vi "specs_prodigy.vi"() -> ()   [LabVIEW 2020]
uses:
  Github/ARPEScontrol/subvi/PHOIBOS/DEFINITIONS/DEF_dev_state.ctl
  Github/ARPEScontrol/subvi/PHOIBOS/DEFINITIONS/DEF_dev_type.ctl
panel:
  in  "stop":bool
  in  "ana_mode":T1(ring)=enum."WideAngleMode"
  in  "ana_voltrange":enum16{"3.5kV", "1.5kV", "400V", "100V", "10V"}(ring)=enum."400V"
  in  "phoib_I_2s":dbl=35.0
  in  "phoib_I_1s":dbl=21.0
  in  "phoib_I_6s":dbl=3200.0
  in  "phoib_I_4s":dbl=4.558
  in  "phoib_I_3s":dbl=-10.0
  in  "phoib_I_5s":dbl=1700.0
  in  "phoib_I_7s":dbl=-30.0
  in  "phoib_I_8s":dbl=0.0039
  in  "phoib_I_9s":dbl
  in  "phoib_I_10s":dbl
  out "phoib_I_4":dbl=4.558 caption="Work Function"
  out "phoib_I_5":dbl=1500.0 caption="Detctor Voltage"
  out "phoib_I_6":dbl=3200.0 caption="Screen Voltage"
  out "phoib_I_3":dbl=-10.0 caption="Coil Current"
  out "phoib_I_2":dbl=35.0 caption="Pass Energy"
  out "phoib_I_1":dbl=21.0 caption="Kinetic Energy"
  out "state":T2=1 items=["Off"=-1, "Standby"=0, "On"=1]
  out "phoib_I_7":dbl=-30.0 caption="Conversion Voltage"
  out "phoib_I_8":dbl=0.0039 caption="FD1"
  out "phoib_I_9":dbl caption="Mesh Front"
  out "phoib_I_10":dbl caption="Mesh Back"
  out "phoib_error":errorcluster
  out "phoib_con?":bool caption="PHOIBOS"
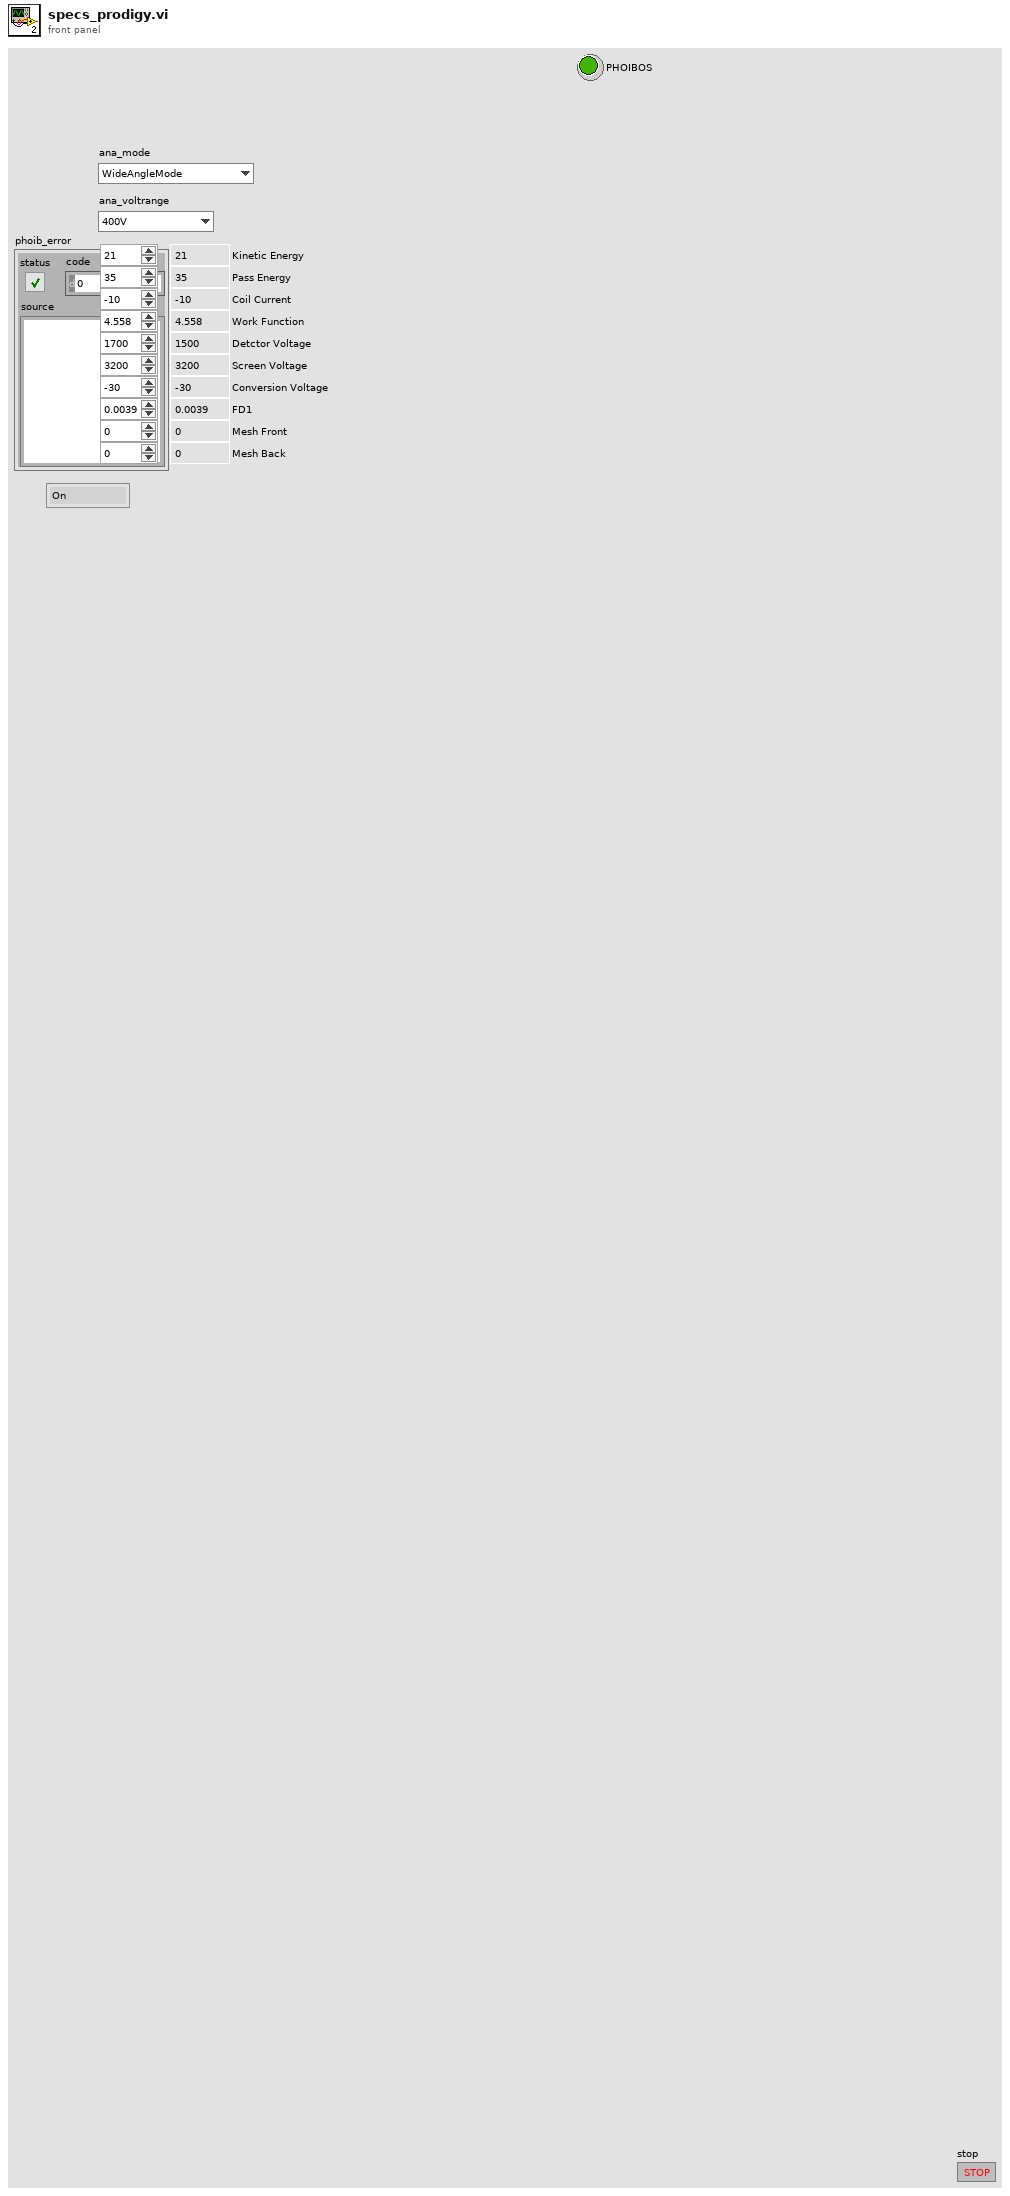
[diagram p1: front panel]
types:
  T1 = enum16{"HighMagnification", "MediumMagnification", "LowMagnification", "HighAngularDispersion", "MediumAngularDispersion", "LowAngularDispersion", "WideAngleMode", "LargeArea", "MediumArea", "SmallArea", "HighMagnification2", "SmallArea2"}
  T2 = typedef "DEF_dev_state.ctl" = i32
  T3 = typedef "DEF_dev_type.ctl" = enum32{"devA (analyzer)", "devD (detector)"}
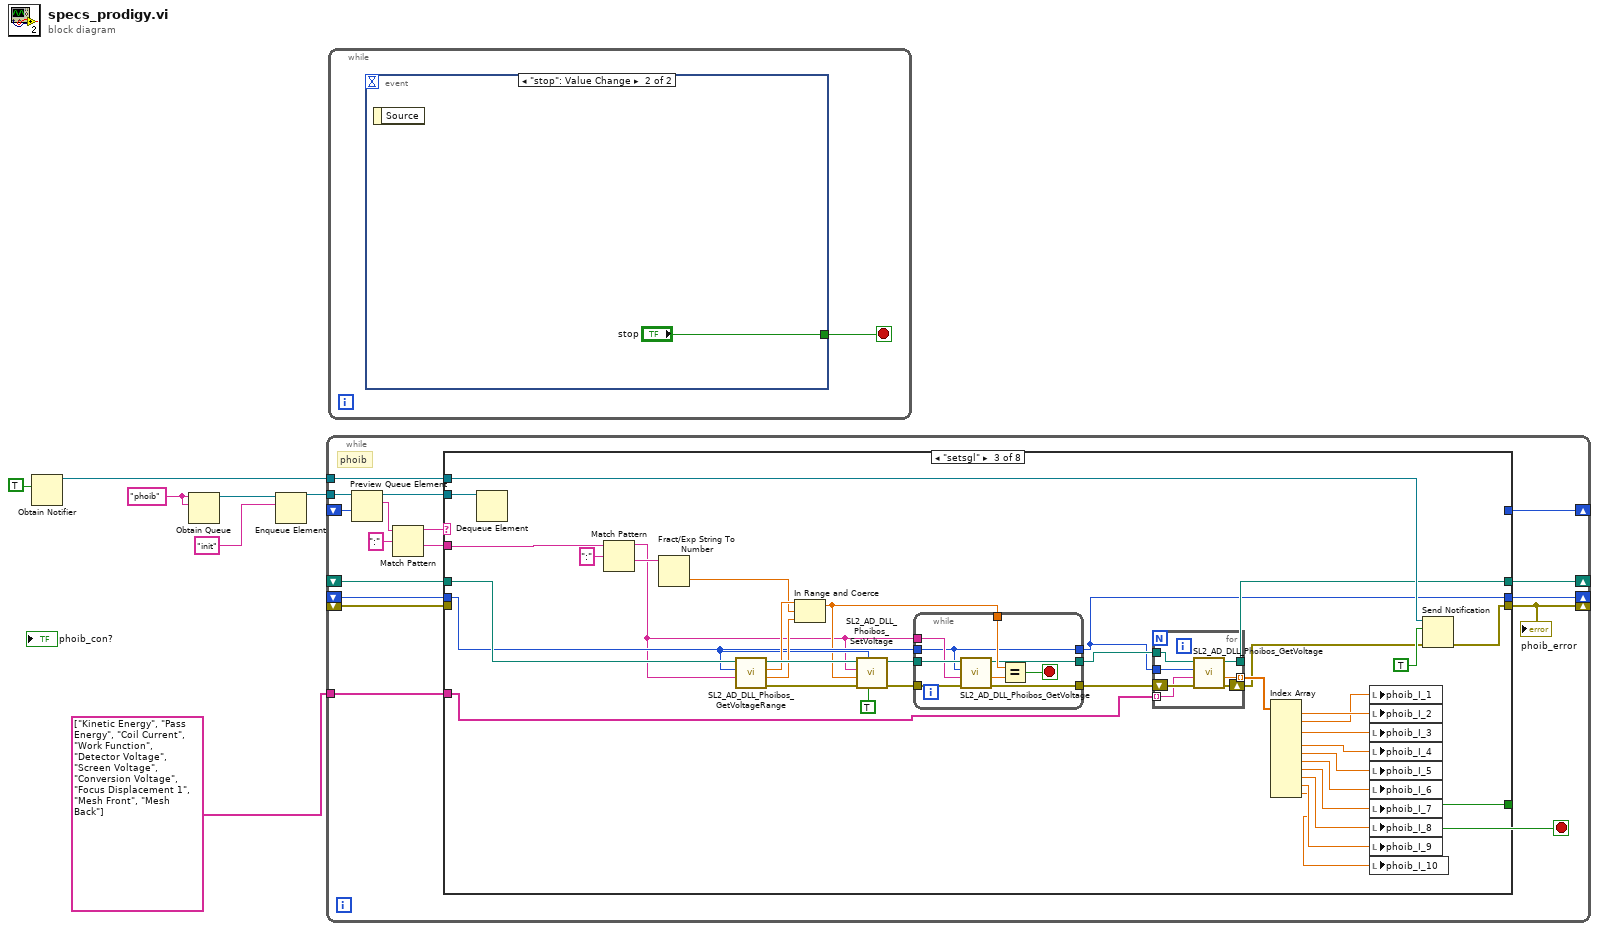
[diagram p0: block diagram]
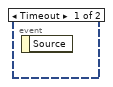
[diagram p2: hidden frame]
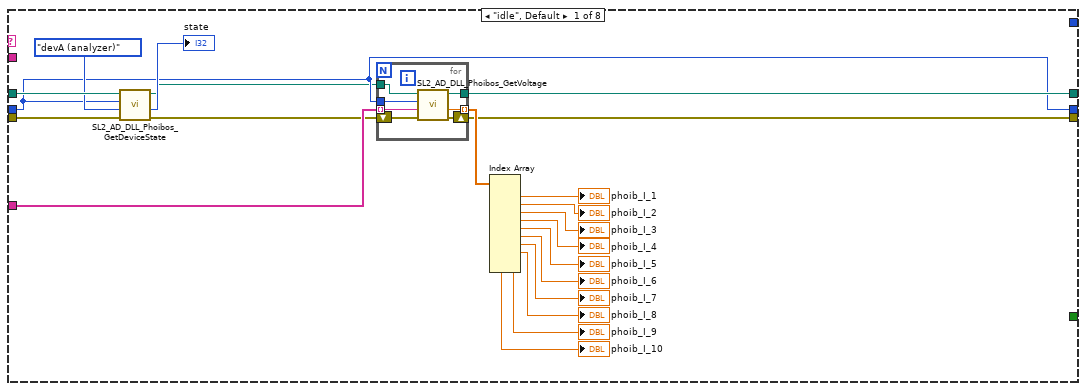
[diagram p3: hidden frame]
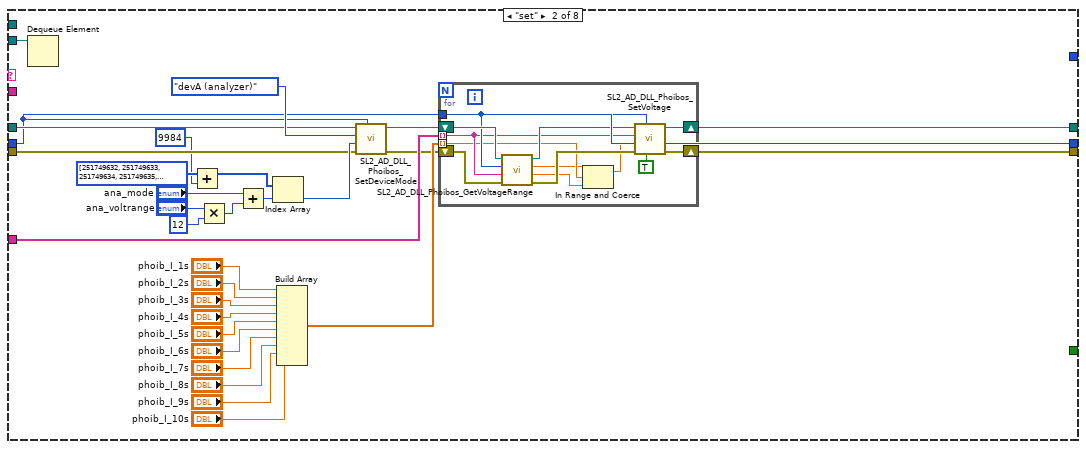
[diagram p4: hidden frame]
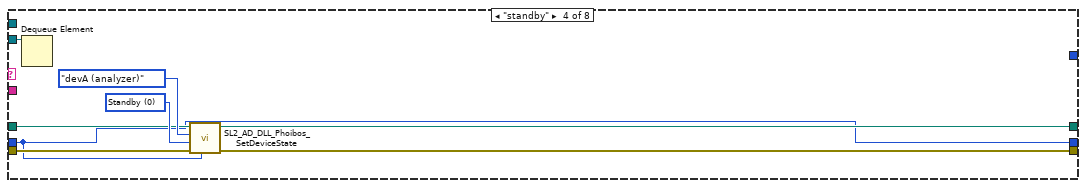
[diagram p5: hidden frame]
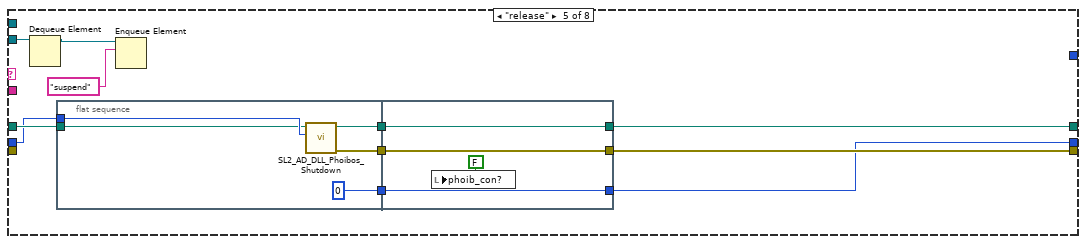
[diagram p6: hidden frame]
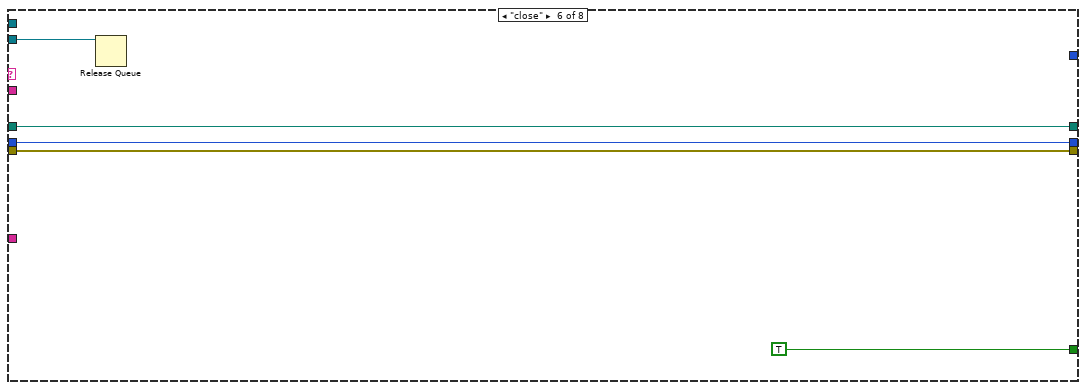
[diagram p7: hidden frame]
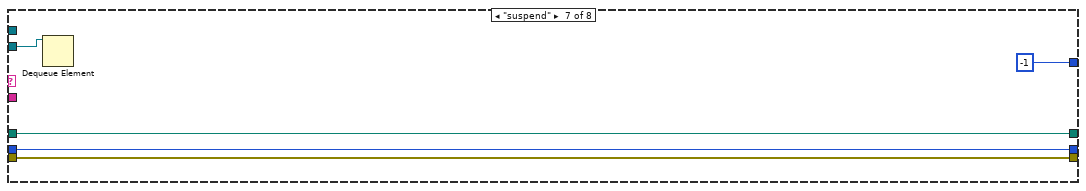
[diagram p8: hidden frame]
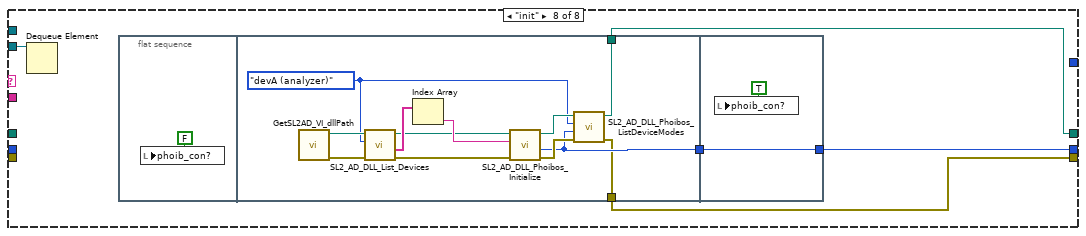
[diagram p9: hidden frame]
diagram:
  w4 = "phoib" ("name (unnamed)")
  n1 = Obtain Notifier(notification data type=TRUE) -> (notifier out=w2:refnum<notifier>)  [unwired: 3 in, 2 out]
  n2 = Obtain Queue(name (unnamed)=w4, element data type=w4) -> (queue out=w7:refnum<queue>)  [unwired: 3 in, 2 out]
  n3 = Enqueue Element(queue=w7, element="init") -> (queue out=w6:refnum<queue>)  [unwired: 2 in, 2 out]
  n4 = while {
    tunnel: w6 -> [w19]
    shift-right: [w8] -> _
    shift-left: _ -> [w17]
    shift-right: [w16] -> _
    shift-left: _ -> [w15]
    shift-right: [w14] -> _
    shift-left: _ -> [w13]
    shift-right: [w12] -> _
    shift-left: _ -> [w11]
    tunnel: string[] ["Kinetic Energy", "Pass Energy", "Coil Current", "Work Function", "Detector Voltage", "Screen Voltage", "Conversion Voltage", "Focus Displacement 1", "Mesh Front", "Mesh Back"] -> [w10]
    tunnel: w2 -> [w9]
    stop <- w18 stop-if-true
    # "phoib"
    n5 = Preview Queue Element(queue=w19, timeout in ms (-1)=w17) -> (queue out=w22:refnum<queue>, element=w23:string)  [unwired: 1 in, 2 out]
    n6 = Match Pattern(string=w23, regular expression=":") -> (before substring=w21:string, after substring=w20:string)  [unwired: 1 in, 2 out]
    n7 = case shown="\"setsgl\"" w21 {
      tunnel: w22 -> [_ w80 w131 w148 w166 w180 w185 w190]
      tunnel: w20 -> [_ _ w96 _ _ _ _ _]
      tunnel: [_ _ _ _ _ TRUE _ _] -> w18
      tunnel: [w34 w82 w101 w151 w164 w178 w184 w187] -> w16
      tunnel: w15 -> [w45 w71 w122 w153 w165 w178 w184 _]
      tunnel: [w33 w81 w117 w150 w163 w176 w182 w186] -> w14
      tunnel: w13 -> [w43 w70 _ w152 _ w176 w182 _]
      tunnel: [w31 w68 w100 w149 w162 w177 w183 w189] -> w12
      tunnel: w11 -> [w31 w68 w120 w149 w161 w177 w183 _]
      tunnel: w10 -> [w32 w61 w98 _ _ _ _ _]
      tunnel: w9 -> [_ _ w116 _ _ _ _ _]
      tunnel: [_ _ _ _ _ _ -1 _] -> w8
      frame "idle", Default {
        n8 = call "SL2_AD_DLL_Phoibos_GetDeviceState.vi"("dll_path"=w45, "pHandle_in"=w31, "dev_type"=DEF_dev_type."devA (analyzer)", "error in"=w43) -> ("path out"=w30:path, "state"=→"state":T2, "error out"=w29:errorcluster)  [unwired: 2 in]
        n9 = for {
          tunnel: w31 -> [w52]
          tunnel: w32 -> [w50] mode=indexing
          tunnel: [w49] -> w42 mode=indexing
          tunnel: [w48] -> w34
          shift-right: [w47] -> w33
          shift-left: w29 -> [w51]
          tunnel: w30 -> [w46]
          n10 = call "SL2_AD_DLL_Phoibos_GetVoltage.vi"("error in"=w51, "voltage_name"=w50, "pHandle"=w52, "dll path in"=w46) -> ("error out"=w47:errorcluster, "value"=w49:dbl, "dll path out"=w48:path)  [unwired: 3 in]
        }
        n11 = Index Array(array=w42) -> (element #1=→"phoib_I_1":dbl, element #2=→"phoib_I_2":dbl, element #3=→"phoib_I_3":dbl, element #4=→"phoib_I_4":dbl, element #5=→"phoib_I_5":dbl, element #6=→"phoib_I_6":dbl, element #7=→"phoib_I_7":dbl, element #8=→"phoib_I_8":dbl, element #9=→"phoib_I_9":dbl, element #10=→"phoib_I_10":dbl)  [unwired: 10 in]
      }
      frame "set" {
        n12 = Dequeue Element(queue=w80) -> ()  [unwired: 2 in, 4 out]
        n13 = Add(x=u32[] [251749632, 251749633, 251749634, 251749635, 251749636, 251749637, 251749638, 251749639, 251749640, 251749641, 251749642, 251749643, 251749644, 251749645, 251749646, 251749647, 251749648, 251749649, 251749650, 251749651, 251749652, 251749653, 251749654, 251749655, 251749656, 251749657, 251749658, 251749659, 251749660, 251749661, 251749662, 251749663, 251749664, 251749665, 251749666, 251749667, 251749668, 251749669, 251749670, 251749671, 251749672, 251749673, 251749674, 251749675, 251749676, 251749677, 251749678, 251749679, 251749680, 251749681, 251749682, 251749683, 251749684, 251749685, 251749686, 251749687, 251749688, 251749689, 251749690, 251749691, 251749692, 251749693, 251749694, 251749695, 251749696] ("modeIDs"), y=9984) -> (x+y=w54:u32[])
        n14 = Multiply(x="ana_voltrange", y=12) -> (x*y=w77:i32)
        n15 = Add(x="ana_mode", y=w77) -> (x+y=w74:i32)
        n16 = Index Array(array=w54, index=w74) -> (element=w72:u32)
        n17 = Build Array("phoib_I_1s", "phoib_I_2s", "phoib_I_3s", "phoib_I_4s", "phoib_I_5s", "phoib_I_6s", "phoib_I_7s", "phoib_I_8s", "phoib_I_9s", "phoib_I_10s") -> (w60:dbl[])
        n18 = call "SL2_AD_DLL_Phoibos_SetDeviceMode.vi"("pHandle"=w68, "error in"=w70, "value"=w72, "dev_type"=DEF_dev_type."devA (analyzer)", "dll path in"=w71) -> ("error out"=w59:errorcluster, "dll path out"=w69:path)  [unwired: 4 in]
        n19 = for {
          tunnel: w68 -> [w88]
          shift-right: [w95] -> w82
          shift-left: w69 -> [w92]
          tunnel: w61 -> [w87] mode=indexing
          tunnel: w60 -> [w86] mode=indexing
          shift-right: [w94] -> w81
          shift-left: w59 -> [w90]
          n20 = call "SL2_AD_DLL_Phoibos_GetVoltageRange.vi"("error in"=w90, "voltage_name"=w87, "pHandle"=w88, "dll path in"=w92) -> ("error out"=w89:errorcluster, "min"=w84:dbl, "max"=w85:dbl, "dll path out"=w91:path)  [unwired: 2 in]
          n21 = In Range and Coerce(upper limit=w85, x=w86, lower limit=w84) -> (coerced(x)=w83:dbl)  [unwired: 1 out]
          n22 = call "SL2_AD_DLL_Phoibos_SetVoltage.vi"("commit"=TRUE, "pHandle"=w88, "error in"=w89, "value"=w83, "voltageName"=w87, "dll path in"=w91) -> ("error out"=w94:errorcluster, "dll path out"=w95:path)  [unwired: 3 in]
        }
      }
      frame "setsgl" {
        n23 = Dequeue Element(queue=w131) -> ()  [unwired: 2 in, 4 out]
        n24 = Match Pattern(string=w96, regular expression=":") -> (before substring=w99:string, after substring=w124:string)  [unwired: 1 in, 2 out]
        n25 = Fract/Exp String To Number(string=w124) -> (number=w123:dbl)  [unwired: 3 in, 1 out]
        n26 = call "SL2_AD_DLL_Phoibos_GetVoltageRange.vi"("voltage_name"=w99, "pHandle"=w120, "dll path in"=w122) -> ("error out"=w128:errorcluster, "min"=w126:dbl, "max"=w127:dbl, "dll path out"=w129:path)  [unwired: 3 in]
        n27 = In Range and Coerce(upper limit=w127, x=w123, lower limit=w126) -> (coerced(x)=w118:dbl)  [unwired: 1 out]
        n28 = call "SL2_AD_DLL_Phoibos_SetVoltage.vi"("commit"=TRUE, "pHandle"=w120, "error in"=w128, "value"=w118, "voltageName"=w99, "dll path in"=w129) -> ("error out"=w119:errorcluster, "dll path out"=w121:path)  [unwired: 3 in]
        n29 = while {
          tunnel: w121 -> [w147]
          tunnel: w120 -> [w141]
          tunnel: w99 -> [w146]
          tunnel: w119 -> [w145]
          tunnel: w118 -> [w144]
          tunnel: [w141] -> w100
          tunnel: [w140] -> w102
          tunnel: [w139] -> w104
          stop <- w142 stop-if-true
          n30 = call "SL2_AD_DLL_Phoibos_GetVoltage.vi"("error in"=w145, "voltage_name"=w146, "pHandle"=w141, "dll path in"=w147) -> ("error out"=w139:errorcluster, "value"=w143:dbl, "dll path out"=w140:path)  [unwired: 3 in]
          n31 = Equal?(x=w144, y=w143) -> (x = y?=w142:bool)
        }
        n32 = for {
          tunnel: w100 -> [w138]
          tunnel: [w136] -> w105 mode=indexing
          tunnel: [w135] -> w101
          shift-right: [w134] -> w103
          shift-left: w104 -> [w137]
          tunnel: w102 -> [w133]
          tunnel: w98 -> [w132] mode=indexing
          n33 = call "SL2_AD_DLL_Phoibos_GetVoltage.vi"("error in"=w137, "voltage_name"=w132, "pHandle"=w138, "dll path in"=w133) -> ("error out"=w134:errorcluster, "value"=w136:dbl, "dll path out"=w135:path)  [unwired: 3 in]
        }
        n34 = Index Array(array=w105) -> (element #1=w106:dbl, element #2=w107:dbl, element #3=w108:dbl, element #4=w109:dbl, element #5=w110:dbl, element #6=w114:dbl, element #7=w111:dbl, element #8=w112:dbl, element #9=w113:dbl, element #10=w97:dbl)  [unwired: 10 in]
        n35 = local write "phoib_I_1"(w106) -> ()
        n36 = local write "phoib_I_2"(w107) -> ()
        n37 = local write "phoib_I_3"(w108) -> ()
        n38 = local write "phoib_I_4"(w109) -> ()
        n39 = local write "phoib_I_5"(w110) -> ()
        n40 = local write "phoib_I_6"(w114) -> ()
        n41 = local write "phoib_I_7"(w111) -> ()
        n42 = local write "phoib_I_8"(w112) -> ()
        n43 = local write "phoib_I_9"(w113) -> ()
        n44 = local write "phoib_I_10"(w97) -> ()
        n45 = Send Notification(notification=TRUE, notifier=w116, error in (no error)=w103) -> (error out=w117:errorcluster)  [unwired: 1 out]
      }
      frame "standby" {
        w154 = T2 0 items=["Off"=-1, "Standby"=0, "On"=1] ("state")
        n46 = Dequeue Element(queue=w148) -> ()  [unwired: 2 in, 4 out]
        n47 = call "SL2_AD_DLL_Phoibos_SetDeviceState.vi"("pHandle_in"=w149, "error in"=w152, "state"=w154, "dev_type"=DEF_dev_type."devA (analyzer)", "dll_path"=w153) -> ("error out"=w150:errorcluster, "path out"=w151:path)  [unwired: 2 in]
      }
      frame "release" {
        n48 = Dequeue Element(queue=w166) -> (queue out=w156:refnum<queue>)  [unwired: 2 in, 3 out]
        n49 = flat-sequence {
          tunnel: w165 -> [w167]
          tunnel: w161 -> [w168]
          tunnel: [w171] -> w160
          tunnel: [w170] -> w159
          tunnel: [u32 0] -> w158
          tunnel: [w173] -> w162
          tunnel: [w174] -> w163
          tunnel: [w175] -> w164
          tunnel: w160 -> [w175]
          tunnel: w159 -> [w174]
          tunnel: w158 -> [w173]
          frame #0 {
            n50 = call "SL2_AD_DLL_Phoibos_Shutdown.vi"("pHandle"=w168, "dll path in"=w167) -> ("error out"=w170:errorcluster, "dll path out"=w171:path)  [unwired: 4 in]
          }
          frame #1 {
            n51 = local write "phoib_con?"(FALSE ("phoib_con?")) -> ()
          }
        }
        n52 = Enqueue Element(queue=w156, element="suspend") -> ()  [unwired: 2 in, 3 out]
      }
      frame "close" {
        n53 = Release Queue(queue=w180) -> ()  [unwired: 2 in, 3 out]
      }
      frame "suspend" {
        n54 = Dequeue Element(queue=w185) -> ()  [unwired: 2 in, 4 out]
      }
      frame "init" {
        n55 = Dequeue Element(queue=w190) -> ()  [unwired: 2 in, 4 out]
        n56 = flat-sequence {
          tunnel: [w197] -> w188
          tunnel: [w193] -> w187
          tunnel: [w192] -> w186
          tunnel: [w205] -> w189
          tunnel: w188 -> [w205]
          frame #0 {
            n57 = local write "phoib_con?"(FALSE ("phoib_con?")) -> ()
          }
          frame #1 {
            w196 = DEF_dev_type."devA (analyzer)" ("dev_type")
            n58 = call "GetSL2AD_VI_dllPath.vi"() -> ("error"=w200:errorcluster, "Path"=w201:path)  [unwired: 9 in, 1 out]
            n59 = call "SL2_AD_DLL_List_Devices.vi"("error in"=w200, "dev_type"=w196, "dll path in"=w201) -> ("error out"=w194:errorcluster, "devices"=w203:string[], "dll path out"=w195:path)  [unwired: 2 in]
            n60 = Index Array(array=w203) -> (element=w202:string)  [unwired: 1 in]
            n61 = call "SL2_AD_DLL_Phoibos_Initialize.vi"("error in"=w194, "analyzerId"=w202, "dll_path"=w195) -> ("error out"=w198:errorcluster, "pHandle"=w197:u32, "path out"=w199:path)  [unwired: 2 in]
            n62 = call "SL2_AD_DLL_Phoibos_ListDeviceModes.vi"("dll path in"=w199, "dev_type"=w196, "pHandle"=w197, "error in"=w198) -> ("dll path out"=w193:path, "error out"=w192:errorcluster)  [unwired: 1 in, 2 out]
          }
          frame #2 {
            n63 = local write "phoib_con?"(TRUE ("phoib_con?")) -> ()
          }
        }
      }
    }
    "phoib_error" <- w14
  }
  n64 = while {
    stop <- w206 stop-if-true
    n65 = event shown="[1] \"stop\": Value Change" {
      selector: _ -> [_ _]
      dyn-events: _ -> [_ _]
      timeout: _ -> [_ _]
      tunnel: [_ "stop"] -> w206
      event Timeout {
        n66 = event-data() -> ()  [unwired: 1 in, 1 out]
      }
      event "stop": Value Change {
        n67 = event-data() -> ()  [unwired: 1 in, 1 out]
      }
    }
  }
